vi "ReadAll.vi"(8 "error in (no error)":errorcluster, 11 "BME680 in":refnum<class "BME680.lvclass">) -> (0 "error out":errorcluster, 1 "Hum":u8, 2 "Pres":u32, 3 "BME680 out":refnum<class "BME680.lvclass">, 5 "Temp":u16)   [LabVIEW 2022 SP3, in "BME680.lvlib" / "BME680.lvclass"]
uses:
  BME680.lvclass
  BME680.lvclass/BME680.ctl
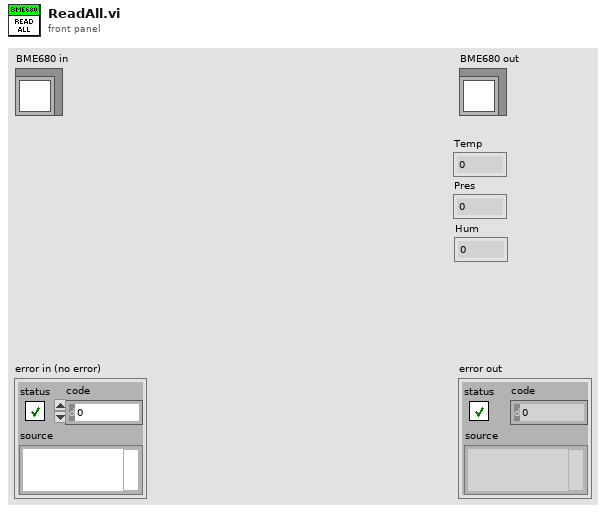
[diagram p1: front panel]
types:
  T1 = typedef "BME680.lvlib/BME680.lvclass/Data.ctl" = cluster{"Status":u8, "GasIdx":u8, "MeasIdx":u8, "ResHeat":u8, "iDac":u8, "GasWait":u8, "Temp":u16, "Pres":u32, "Hum":u8, "Gas Res":u8}
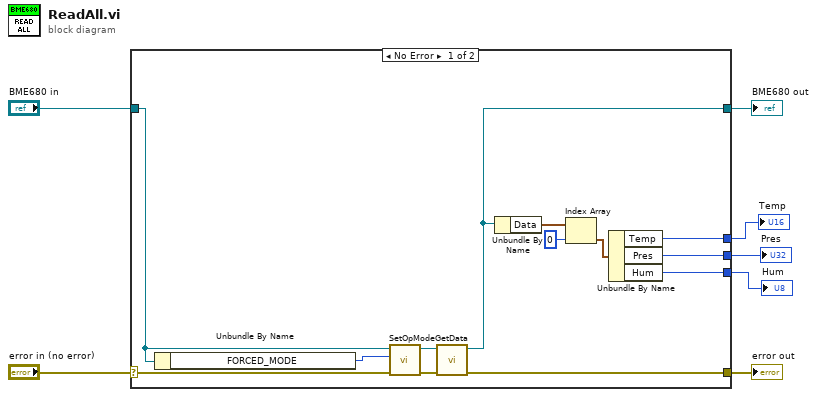
[diagram p0: block diagram]
diagram:
  n1 = case shown="No Error" "error in (no error)" {
    selector: "error in (no error)" -> [w18 w22]
    tunnel: [w20 w22] -> w6
    tunnel: [w19 w21] -> w4
    tunnel: "BME680 in" -> [w15 w21]
    tunnel: [w10 _] -> w3
    tunnel: [w9 _] -> w2
    tunnel: [w8 _] -> w1
    frame No Error {
      n2 = Unbundle By Name(w15) -> ("FORCED_MODE"=w14:u8)
      n3 = call-dynamic "SetOpMode.vi"("error in (no error)"=w18, "Op Mode"=w14, "BME680 in"=w15) -> ("error out"=w17:errorcluster, "BME680 out"=w16:refnum<class "BME680.lvclass">)  [unwired: 7 in]
      n4 = call-dynamic "GetData.vi"("error in (no error)"=w17, "BME68x in"=w16) -> ("error out"=w20:errorcluster, "BME68x out"=w19:refnum<class "BME680.lvclass">)  [unwired: 8 in]
      n5 = Unbundle By Name(w19) -> ("Data"=w13:T1[])
      n6 = Index Array(array=w13, index=0) -> (element=w11:T1)
      n7 = Unbundle By Name(w11) -> ("Temp"=w10:u16, "Pres"=w9:u32, "Hum"=w8:u8)
    }
    frame Error {
    }
  }
  "error out" <- w6
  "BME680 out" <- w4
  "Temp" <- w3
  "Pres" <- w2
  "Hum" <- w1
